vi "UsrProfiles-Refresh profiles list after name edit.vi"(8 "error in":errorcluster) -> (0 "error out":errorcluster)   [LabVIEW 2017]
uses:
  Typedefs/Save-Load enum.ctl
  Globals/gl_UsrProfiles globals.vi
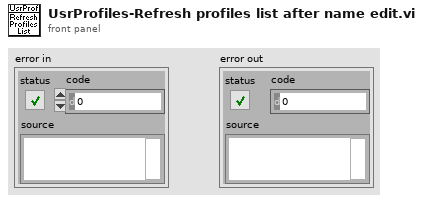
[diagram p1: front panel]
types:
  T1 = typedef "Save-Load enum.ctl" = enum16{"Save to file", "Load from file", "Compare from file"}
  T2 = typedef "User login window refs.ctl" = cluster{"User profiles window ref":refnum<k9>, "Users listbox":refnum<vi>, "Profiles listbox":refnum<vi>, "Last used":refnum<vi>}
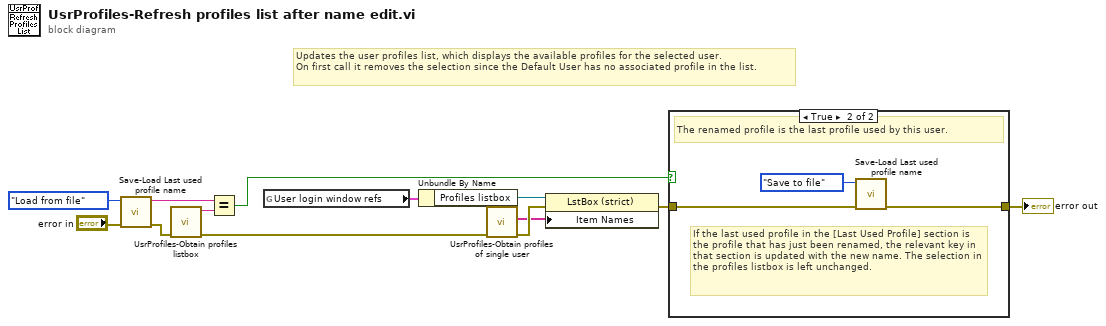
[diagram p0: block diagram]
diagram:
  # "Updates the user profiles list, which displays the available profiles for the selected user.\nOn first call it removes the selection since the Default User has no associated profile in the list."
  n1 = call "Save-Load Last used profile name.vi"("error in"="error in", "Function"=Save-Load_enum."Load from file") -> ("error out"=w9:errorcluster, "Last used profile for selected user"=w12:string)  [unwired: 7 in, 1 out]
  n2 = call "UsrProfiles-Obtain profiles listbox.vi"("error in (no error)"=w9) -> ("error out"=w3:errorcluster, "Selected profile's name"=w10:string)  [unwired: 7 in, 2 out]
  n3 = Equal?(x=w12, y=w10) -> (x = y?=w11:bool)
  n4 = global read "gl_UsrProfiles globals.vi" "User login window refs"() -> (w4:T2)
  n5 = Unbundle By Name(w4) -> ("Profiles listbox"=w5:refnum<vi>)
  n6 = call "UsrProfiles-Obtain profiles of single user.vi"("error in"=w3) -> ("error out"=w7:errorcluster, "User profile names"=w6:string[])  [unwired: 9 in]
  n7 = property on="Property Node" class="LstBox (strict)"(reference=w5, error in=w7, "Item Names"=w6) -> (error out=w2:errorcluster)  [unwired: 1 out]
  n8 = case shown="True" w11 {
    tunnel: [w14 w16] -> w8
    tunnel: w2 -> [w14 w15]
    frame False {
    }
    frame True {
      # "If the last used profile in the [Last Used Profile] section is the profile that has just been renamed, the relevant key in that section is updated with the new name. The selection in the profiles listbox is left unchanged."
      # "The renamed profile is the last profile used by this user."
      n9 = call "Save-Load Last used profile name.vi"("error in"=w15, "Function"=Save-Load_enum."Save to file") -> ("error out"=w16:errorcluster)  [unwired: 7 in, 2 out]
    }
  }
  "error out" <- w8
